vi "Main.vi"() -> ()   [LabVIEW 2014, in "Folder Shot.lvlib"]
uses:
  Folder Shot.lvlib
  Source/SLL File IO/_Typedefs/Folder Shot Result.ctl
  <vilib>/Utility/error.llb/DialogType.ctl
  Source/SLL Queued State Machine/Queue Driver/Create Queue.vi
  Source/SLL Queued State Machine/Queue Driver/Enqueue an Item to Queue.vi
  Source/SLL Queued State Machine/Queue Driver/Dequeue Queue.vi
  Source/SLL Queued State Machine/Queue Driver/Enqueue N Items.vi
  Source/SLL Queued State Machine/Queue Driver/Flush Queue.vi
  Source/SLL Queued State Machine/Queue Driver/Release Queue.vi
  Source/SLL Queued State Machine/SLL QSM.lvlib
  Source/SLL File IO/SLL File IO.lvlib
  Source/SLL String/SLL String.lvlib
panel:
  in  "Save Result":bool
  out "Status":string
  out "Added":i32
  out "Deleted":i32
  out "Modified":i32
  out "Folder Shot Results":T1
  in  "Run":bool
  in  "Tab Control":T2(tab)
  in  "Compare Folders":cluster{"Folder 1":path, "Folder 2":path}
  in  "Compare Folder Shots":T3
  in  "Folder Shot Report Folder":path
  in  "Folder Path":path
  in  "Folders to Exclude[]":string[](array[string])=[".git", ".svn"]
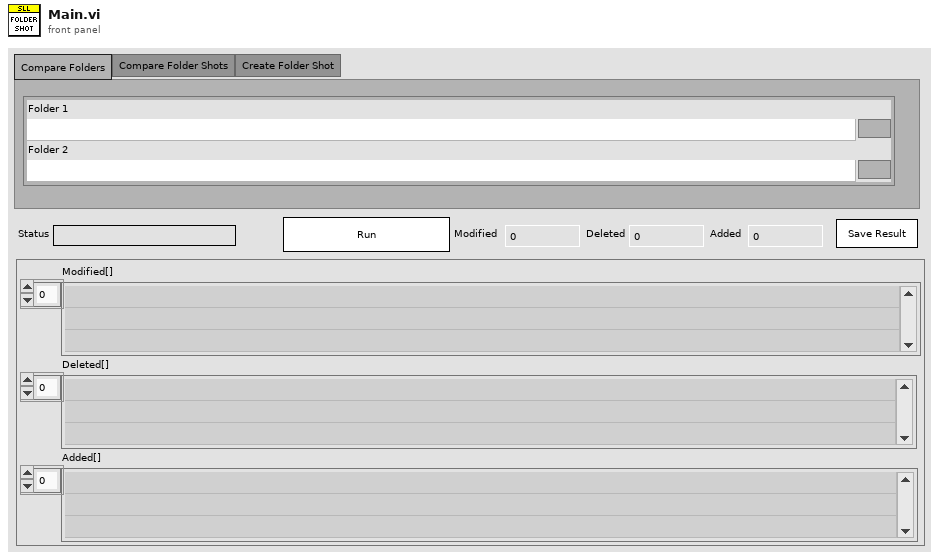
[diagram p1: front panel]
types:
  T1 = typedef "SLL File IO.lvlib/Folder Shot Result.ctl" = cluster{"Modified[]":path[], "Deleted[]":path[], "Added[]":path[]}
  T2 = enum32{"Compare Folders", "Compare Folder Shots", "Create Folder Shot"}
  T3 = cluster{"Folder Shot 1":path, "Folder Shot 2":path}
  T4 = cluster{"Flags":cluster{"Source Code?":bool}, "Folder Shot Results":T1}
  T5 = typedef "DialogType.ctl" = u16
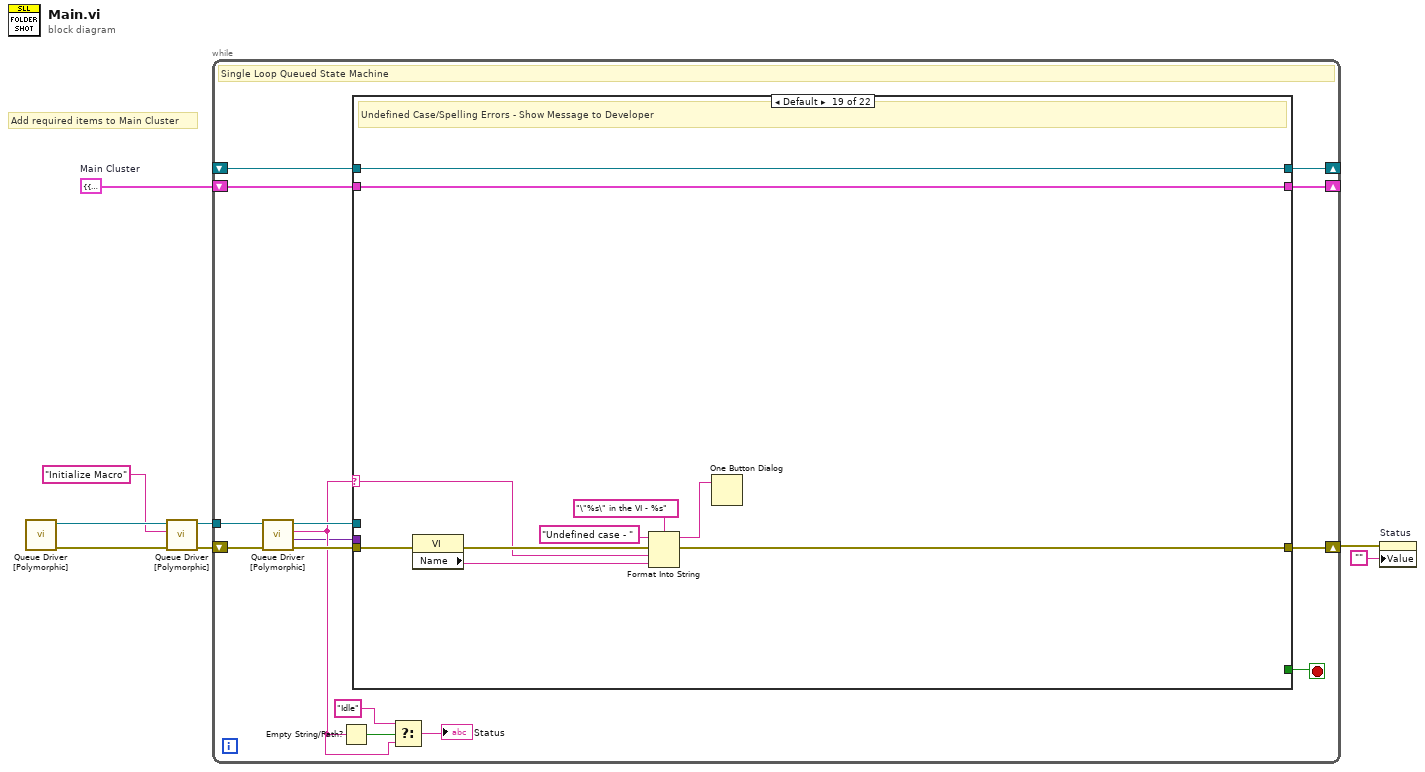
[diagram p0: block diagram]
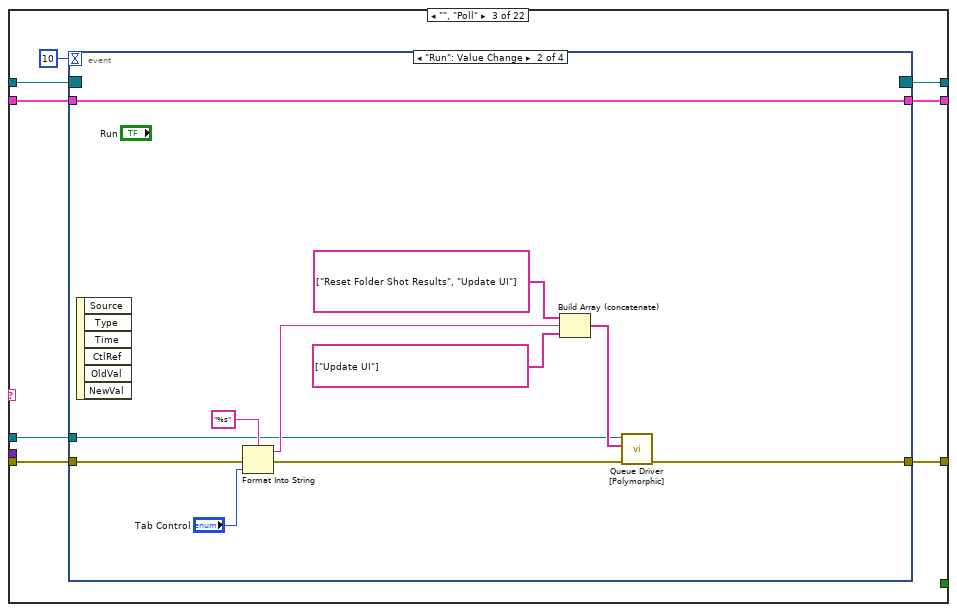
[diagram p4: hidden frame]
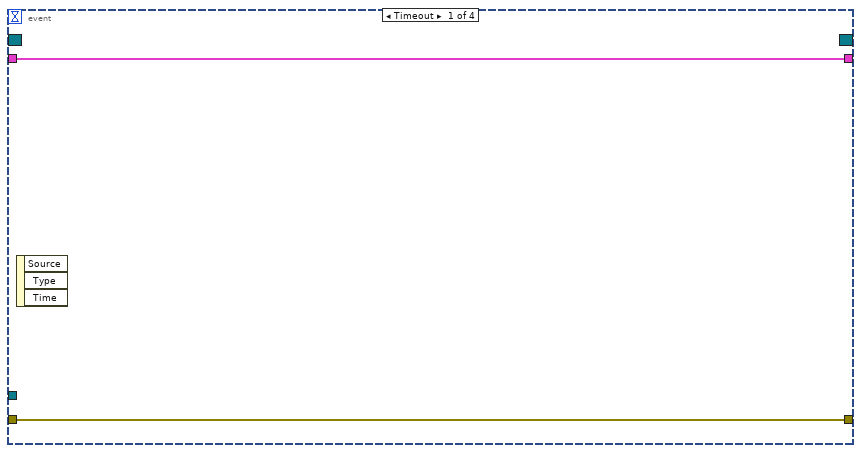
[diagram p5: hidden frame]
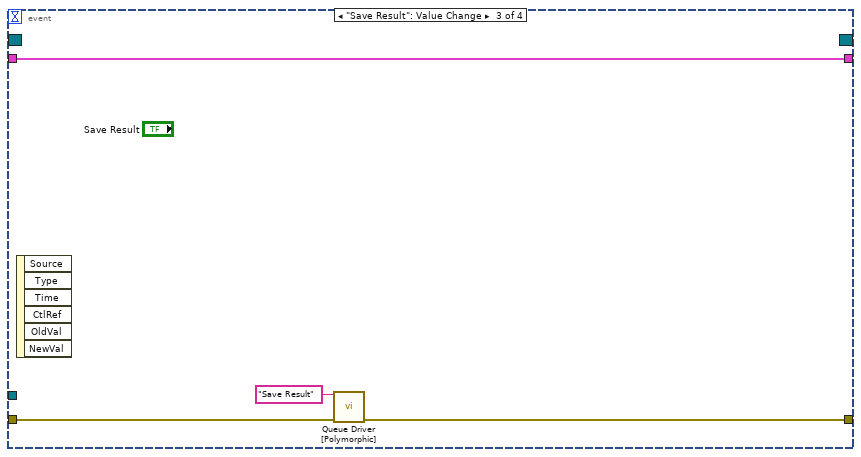
[diagram p6: hidden frame]
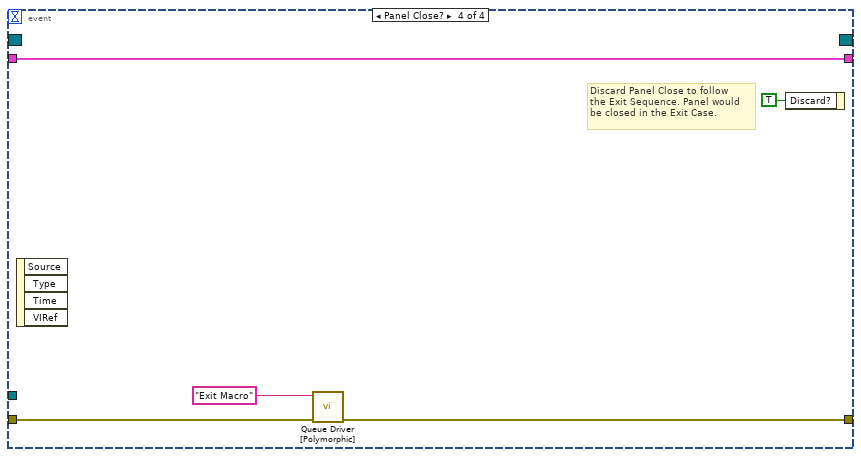
[diagram p7: hidden frame]
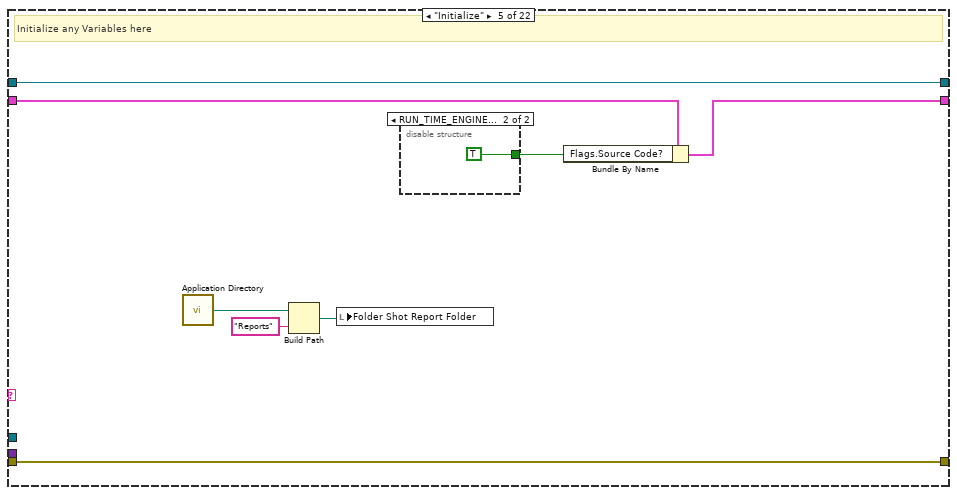
[diagram p9: hidden frame]
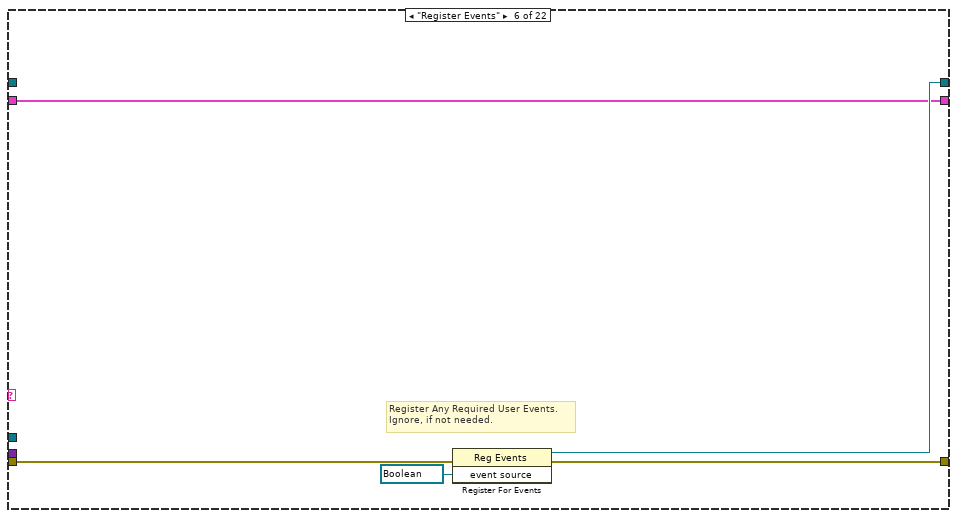
[diagram p11: hidden frame]
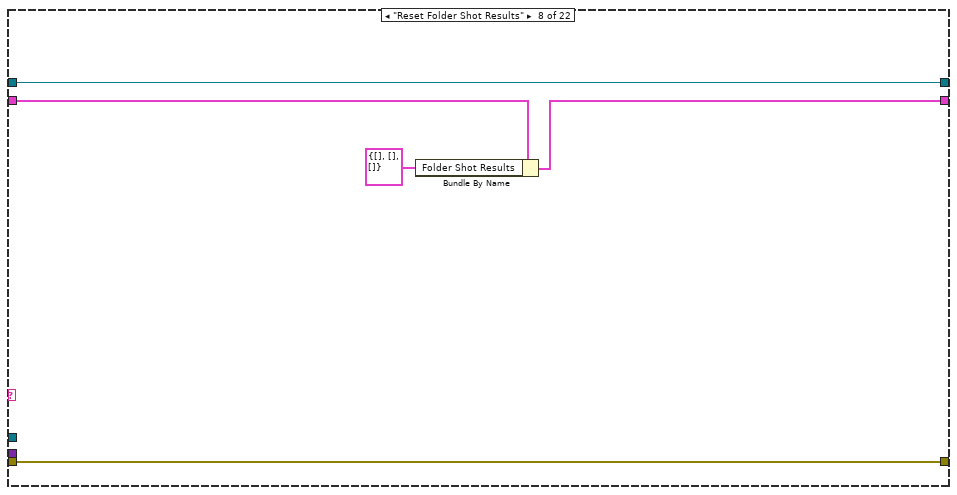
[diagram p13: hidden frame]
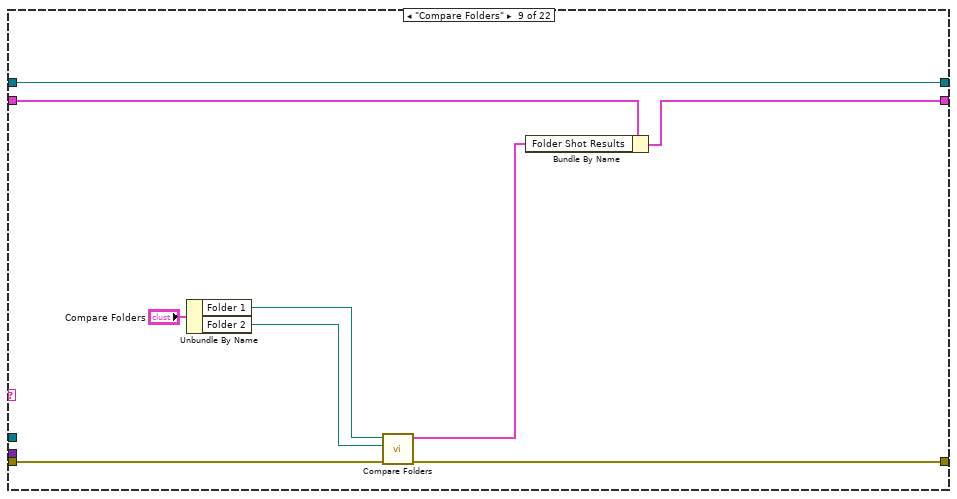
[diagram p14: hidden frame]
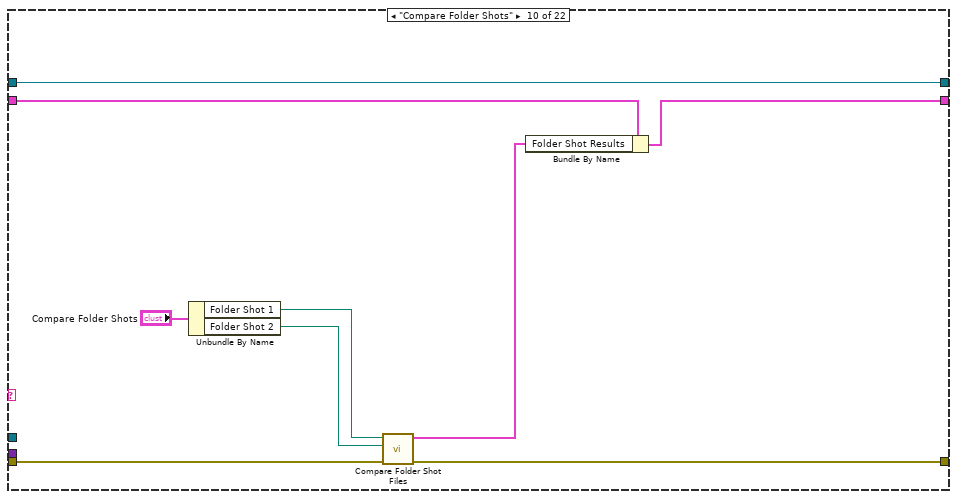
[diagram p15: hidden frame]
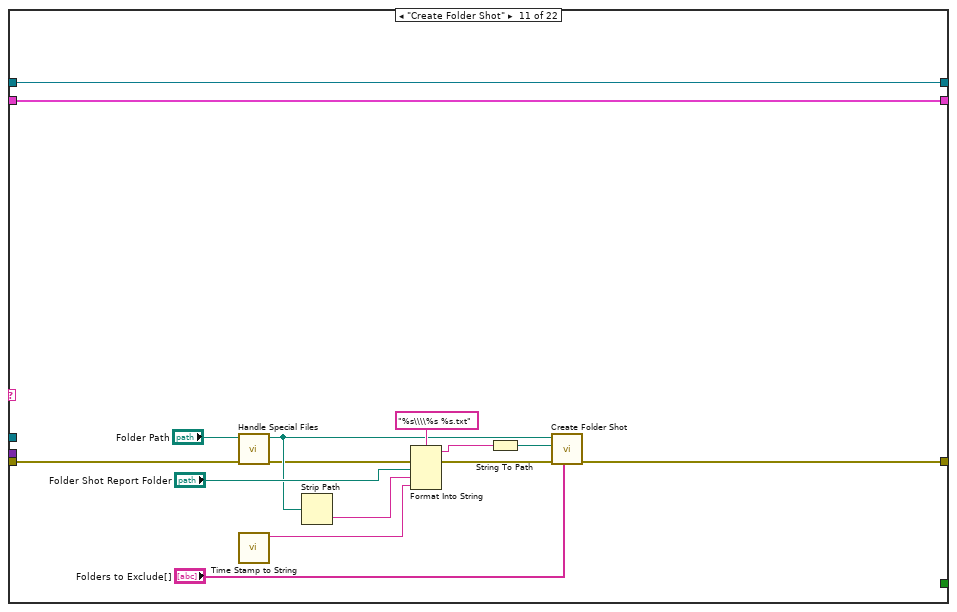
[diagram p16: hidden frame]
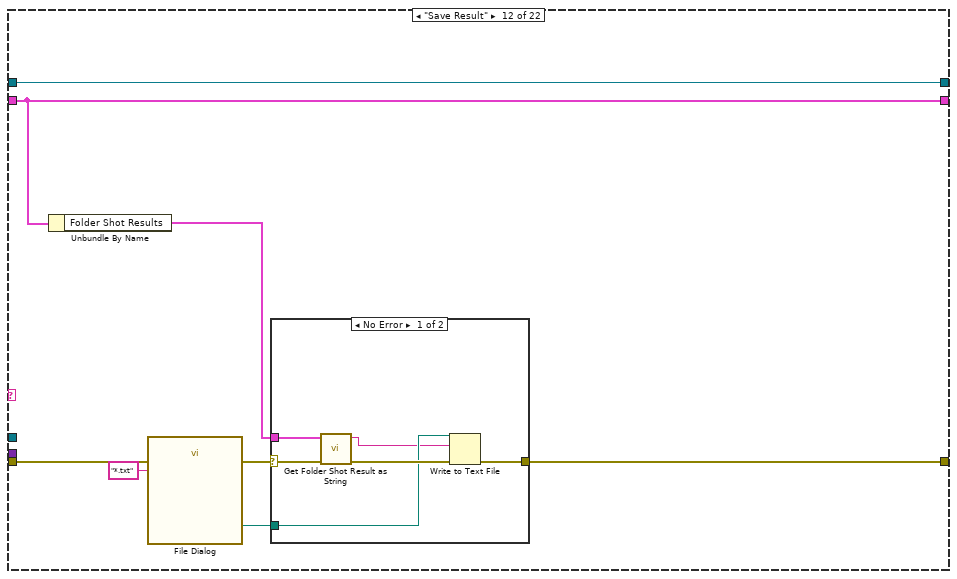
[diagram p17: hidden frame]
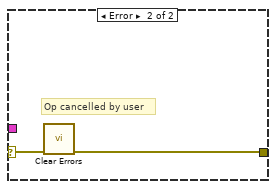
[diagram p18: hidden frame]
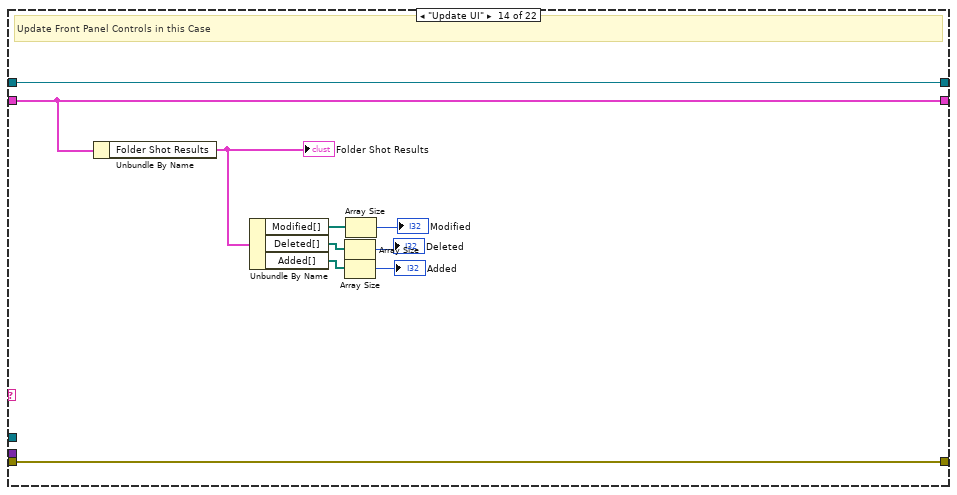
[diagram p20: hidden frame]
diagram:
  w8 = T4 {"Flags"={"Source Code?"=FALSE}, "Folder Shot Results"={"Modified[]"=[], "Deleted[]"=[], "Added[]"=[]}}  # Main Cluster
  # "Add required items to Main Cluster"
  n1 = call-poly "Queue Driver [Polymorphic].vi"() -> ("Error Out"=w6:errorcluster, "Queue Ref"=w3:refnum<queue>)  [unwired: 10 in]
  n2 = call-poly "Queue Driver [Polymorphic].vi"("Error In"=w6, "Item to Add"="Initialize Macro", "Queue Ref In"=w3) -> ("Error Out"=w7:errorcluster, "Queue Ref Out"=w1:refnum<queue>)  [unwired: 7 in]
  n3 = while "SLL Queued State Machine" {
    shift-right: [w21] -> w5
    shift-left: w7 -> [w23]
    shift-right: [w19] -> _
    shift-left: _ -> [w18]
    shift-right: [w17] -> _
    shift-left: w8 -> [w16]
    tunnel: w1 -> [w9]
    stop <- w20 stop-if-true
    # "Single Loop Queued State Machine"
    n4 = call-poly "Queue Driver [Polymorphic].vi"("Error In"=w23, "Queue Ref In"=w9) -> ("Error Out"=w22:errorcluster, "Data"=w10:variant, "Dequeue"=w11:string, "Queue Ref Out"=w14:refnum<queue>)  [unwired: 6 in]
    n5 = Empty String/Path?(string/path=w11) -> (empty?=w15:bool)
    n6 = case "QSM Case Structure" shown="Default" w11 {
      selector: w11 -> [_ _ _ _ _ _ _ _ _ _ _ _ _ _ _ _ _ _ w165 _ _ _]
      tunnel: w22 -> [w26 w29 w35 w62 w70 w76 w79 w84 w93 w102 w103 w125 w136 w146 w149 w153 w159 w164 w168 w180 w183 w196]
      tunnel: [w26 w29 w36 w62 w70 w75 w79 w84 w89 w99 w115 w119 w136 w146 w149 w152 w158 w164 w171 w178 w183 w192] -> w21
      tunnel: [_ _ _ _ _ _ _ _ _ _ _ _ _ _ _ _ _ _ _ _ _ TRUE] -> w20
      tunnel: [w25 w28 w34 w61 w69 w74 w78 w83 w92 w101 w117 w124 w135 w145 w148 w155 w161 w163 w174 w177 w182 w195] -> w19
      tunnel: w18 -> [w25 w28 w33 w61 w69 _ w78 w83 w92 w101 w117 w124 w135 w145 w148 w155 w161 w163 w174 w177 w182 w195]
      tunnel: [w24 w27 w31 w60 w66 w73 w77 w81 w86 w96 w116 w121 w134 w144 w147 w154 w160 w162 w173 w176 w181 w194] -> w17
      tunnel: w16 -> [w24 w27 w32 w60 w67 w73 w77 w82 w91 w100 w116 w121 w134 w144 w147 w154 w160 w162 w173 w176 w181 w194]
      tunnel: w14 -> [_ _ w30 _ _ _ _ _ _ _ _ _ _ _ _ w151 w156 _ _ _ _ w185]
      tunnel: w10 -> [_ _ _ _ _ _ _ _ _ _ _ _ _ _ _ _ _ _ _ _ _ _]
      frame "/--------------- Read Me -----------------/" {
        # "General Purpose Queue Based State Machine for Any Use Case (main application, module, pop up message etc)\n\nAdvantages:\n1. No Need to Pass Queue References between Queue Driver VIs.\n2. This template can be safely used in multiple parallel running modules without any issues.\n3. This template can also be safely used even in cases where the VI is configured to be a Clone, where multiple \ninstances of the VI could be executing concurrently.\n\nHow to Use:\n1. Add necessary items to the Main Cluster.\n2. Use the Polymorphic Queue Driver for doing any queue operations. There is no need to pass the queue driver\nreference, as the Queue Driver automatically infers the reference based on the VI instance from which it is called.\n3. Add any required user events in the \"Register Events\" case. Ignore if not needed.\n4. Use \"Sequences\" section for defining any list of state calls, which could be used in multiple places. \nEg: Initialize Sequence, might be needed if we need to any reinitialization."
      }
      frame "/------------------ Poll -------------------/" {
      }
      frame "", "Poll" {
        n7 = event shown="[1] \"Run\": Value Change" {
          selector: w33 -> [_ _ _ _]
          dyn-events: [_ _ _ _] -> w34
          timeout: 10 -> [_ _ _ _]
          tunnel: [w39 w45 w53 w58] -> w36
          tunnel: w35 -> [w39 w50 w52 w59]
          tunnel: w32 -> [w38 w49 w54 w57]
          tunnel: [w38 w49 w54 w57] -> w31
          tunnel: w30 -> [_ w40 _ _]
          event Timeout {
            n8 = event-data() -> ()  [unwired: 1 in, 3 out]
          }
          event "Run": Value Change {
            n9 = event-data() -> ()  [unwired: 1 in, 6 out]
            n10 = Format Into String(format string="%s", error in=w50, "Tab Control") -> (resulting string=w42:string, error out=w46:errorcluster)  [unwired: 1 in]
            n11 = Build Array (concatenate)(string[] ["Reset Folder Shot Results", "Update UI"] ("Enqueue N"), w42, string[] ["Update UI"] ("Enqueue N")) -> (w41:string[])
            n12 = call-poly "Queue Driver [Polymorphic].vi"("Error In"=w46, "Enqueue N"=w41, "Queue Ref In"=w40) -> ("Error Out"=w45:errorcluster)  [unwired: 7 in, 1 out]
          }
          event "Save Result": Value Change {
            n13 = event-data() -> ()  [unwired: 1 in, 6 out]
            n14 = call-poly "Queue Driver [Polymorphic].vi"("Error In"=w52, "Queue Name (Optional)"="Save Result" ("Item to Add")) -> ("Error Out"=w53:errorcluster)  [unwired: 8 in, 1 out]
          }
          event Panel Close? {
            # "Discard Panel Close to follow\nthe Exit Sequence. Panel would\nbe closed in the Exit Case."
            n15 = event-data() -> ()  [unwired: 1 in, 4 out]
            n16 = call-poly "Queue Driver [Polymorphic].vi"("Error In"=w59, "Queue Name (Optional)"="Exit Macro" ("Enqueue")) -> ("Error Out"=w58:errorcluster)  [unwired: 8 in, 1 out]
            n17 = event-data("Discard?"=TRUE) -> ()  [unwired: 1 in, 1 out]
          }
        }
      }
      frame "/--------------- Initialize -----------------/" {
      }
      frame "Initialize" {
        # "Initialize any Variables here"
        n18 = call <vilib>:"Application Directory.vi"() -> ("Application Directory"=w65:path)
        n19 = Build Path(base path=w65, name or relative path="Reports") -> (appended path=w63:path)
        n20 = local write "Folder Shot Report Folder"(w63) -> ()
        n21 = disable-structure shown="RUN_TIME_ENGINE==False" {
          disable-tunnel: [_ TRUE] -> w68
          frame condition #0 {
          }
          frame condition #1 (active) {
          }
        }
        n22 = Bundle By Name(cluster=w67, "Flags.Source Code?"=w68) -> (w66:T4)
      }
      frame "Register Events" {
        # "Register Any Required User Events. \nIgnore, if not needed."
        n23 = register-events(error in=w76, refnum<vi> refnum ("event source")) -> (reference out=w74:refnum<event-registration>, error out=w75:errorcluster)  [unwired: 1 in]
      }
      frame "/---------- Custom Case Splitter ----------/" {
      }
      frame "Reset Folder Shot Results" {
        n24 = Bundle By Name(cluster=w82, "Folder Shot Results"=T1 {"Modified[]"=[], "Deleted[]"=[], "Added[]"=[]}) -> (w81:T4)
      }
      frame "Compare Folders" {
        n25 = Unbundle By Name("Compare Folders") -> ("Folder 1"=w88:path, "Folder 2"=w87:path)
        n26 = call "Compare Folders.vi"("error in (no error)"=w93, "Folder 2"=w87, "Folder 1"=w88) -> ("error out"=w89:errorcluster, "Folder Shot Results"=w85:T1)  [unwired: 7 in]
        n27 = Bundle By Name(cluster=w91, "Folder Shot Results"=w85) -> (w86:T4)
      }
      frame "Compare Folder Shots" {
        n28 = Unbundle By Name("Compare Folder Shots") -> ("Folder Shot 1"=w98:path, "Folder Shot 2"=w97:path)
        n29 = call "Compare Folder Shot Files.vi"("error in (no error)"=w102, "Folder Shot File 2"=w97, "Folder Shot File 1"=w98) -> ("error out"=w99:errorcluster, "Folder Shot Results"=w95:T1)  [unwired: 7 in]
        n30 = Bundle By Name(cluster=w100, "Folder Shot Results"=w95) -> (w96:T4)
      }
      frame "Create Folder Shot" {
        n31 = call "Handle Special Files.vi"("error in (no error)"=w103, "Path In"="Folder Path") -> ("error out"=w104:errorcluster, "Path Out"=w105:path)  [unwired: 8 in]
        n32 = call "Time Stamp to String.vi"() -> ("Output String"=w109:string)  [unwired: 10 in, 1 out]
        n33 = Strip Path(path=w105) -> (name=w108:string)  [unwired: 1 out]
        n34 = Format Into String(format string="%s\\\\%s %s.txt", error in=w104, "Folder Shot Report Folder", w108, w109) -> (resulting string=w107:string, error out=w112:errorcluster)  [unwired: 1 in]
        n35 = String To Path(string=w107) -> (path=w106:path)
        n36 = call "Create Folder Shot.vi"("Folders to Exclude"="Folders to Exclude[]", "error in (no error)"=w112, "Log File Path (*.txt)"=w106, "Directory Path"=w105) -> ("error out"=w115:errorcluster)  [unwired: 6 in, 1 out]
      }
      frame "Save Result" {
        n37 = Unbundle By Name(w121) -> ("Folder Shot Results"=w120:T1)
        n38 = call "File Dialog"("error in"=w125, "pattern (all files)"="*.txt") -> ("selected path"=w118:path, "error out"=w123:errorcluster)  [unwired: 10 in, 2 out]
        n39 = case shown="No Error" w123 {
          selector: w123 -> [w131 w133]
          tunnel: w120 -> [w129 _]
          tunnel: [w128 w132] -> w119
          tunnel: w118 -> [w127 _]
          frame No Error {
            n40 = call "Get Folder Shot Result as String.vi"("error in (no error)"=w131, "Folder Shot Result"=w129) -> ("error out"=w130:errorcluster, "Folder Shot Result"=w126:string)  [unwired: 8 in]
            n41 = Write to Text File(file (use dialog)=w127, text=w126, error in=w130) -> (error out=w128:errorcluster)  [unwired: 1 in, 2 out]
          }
          frame Error {
            # "Op cancelled by user"
            n42 = call <vilib>:"Clear Errors.vi"("error in (no error)"=w133) -> ("error out"=w132:errorcluster)  [unwired: 5 in, 1 out]
          }
        }
      }
      frame "/-------------- User Interface --------------/" {
        # "Duplicate this case to create additional case splitters for readability"
      }
      frame "Update UI" {
        # "Update Front Panel Controls in this Case"
        n43 = Unbundle By Name(w144) -> ("Folder Shot Results"=w143:T1)
        "Folder Shot Results" <- w143
        n44 = Unbundle By Name(w143) -> ("Modified[]"=w142:path[], "Deleted[]"=w141:path[], "Added[]"=w140:path[])
        n45 = Array Size(array=w141) -> (size(s)=→"Deleted":i32)
        n46 = Array Size(array=w140) -> (size(s)=→"Added":i32)
        n47 = Array Size(array=w142) -> (size(s)=→"Modified":i32)
      }
      frame "/----------------- Macros -----------------/" {
      }
      frame "Initialize Macro" {
        w150 = string[] ["Initialize", "Register Events", "Update UI"]  # Initialize Macro
        n48 = call-poly "Queue Driver [Polymorphic].vi"("Error In"=w153, "Enqueue N"=w150, "Queue Ref In"=w151) -> ("Error Out"=w152:errorcluster)  [unwired: 7 in, 1 out]
      }
      frame "Exit Macro" {
        n49 = call-poly "Queue Driver [Polymorphic].vi"("Error In"=w159, "Enqueue N"=string[] ["Exit"], "Queue Ref In"=w156) -> ("Error Out"=w158:errorcluster)  [unwired: 7 in, 1 out]
      }
      frame "/-------------- Error Handler--------------/" {
      }
      frame Default {
        # "Undefined Case/Spelling Errors - Show Message to Developer"
        n50 = property class="VI"(error in=w168) -> (error out=w167:errorcluster, "Name"=w166:string)  [unwired: 1 in, 1 out]
        n51 = Format Into String(format string="\"%s\" in the VI - %s" ("message"), initial string="Undefined case - ", error in=w167, w165, w166) -> (resulting string=w169:string, error out=w171:errorcluster)
        n52 = One Button Dialog(message=w169) -> ()  [unwired: 1 in, 1 out]
      }
      frame "Error" {
        w175 = T5 2 items=["no dialog", "OK message", "continue or stop message", "OK message + warnings", "continue/stop + warnings"] ("type of dialog (OK msg:1)")
        # "Handle the Error"
        n53 = call <vilib>:"Simple Error Handler.vi"("type of dialog (OK msg:1)"=w175, "error in (no error)"=w180) -> ("error out"=w179:errorcluster)  [unwired: 3 in, 4 out]
        n54 = call <vilib>:"Clear Errors.vi"("error in (no error)"=w179) -> ("error out"=w178:errorcluster)  [unwired: 5 in, 1 out]
      }
      frame "/------------------- Exit --------------------/" {
      }
      frame "Exit" {
        n55 = call-poly "Queue Driver [Polymorphic].vi"("Error In"=w196, "Queue Ref In"=w185) -> ("Error Out"=w197:errorcluster, "Queue Ref Out"=w184:refnum<queue>)  [unwired: 7 in, 1 out]
        n56 = Unbundle By Name(w194) -> ("Flags.Source Code?"=w187:bool)
        n57 = call-poly "Queue Driver [Polymorphic].vi"("Error In"=w197, "Queue Ref In"=w184) -> ("Error Out"=w193:errorcluster)  [unwired: 9 in]
        n58 = Call Chain() -> (call chain=w191:string[])
        n59 = Array Size(array=w191) -> (size(s)=w190:i32)
        n60 = Equal?(x=w190, y=1) -> (x = y?=w188:bool)
        n61 = And(x=w187, y=w188) -> (x .and. y?=w186:bool)
        n62 = case "Skip Panel Close when in Source\nCode and is the top most caller" shown="True" w186 {
          tunnel: w193 -> [w200 w202]
          tunnel: [w201 w202] -> w192
          frame False {
            # "Close Panel"
            n63 = invoke class="VI" method="FP.Close"() -> (error out=w199:errorcluster)  [unwired: 3 in, 2 out]
            n64 = Merge Errors(w200, w199) -> (w201:errorcluster)
          }
          frame True {
            # "Do Not Close Panel"
          }
        }
      }
    }
    n65 = Select(t="Idle", s=w15, f=w11) -> (s? t:f=→"Status":string)
  }
  n66 = property on="Status" class="Str"(error in=w5, "Value"="") -> ()  [unwired: 1 in, 2 out]
